vi "Test_Read.vi"   [LabVIEW 2019, in "Test_Maui.Config.lvclass"]
uses:
  Test_Maui.Config.lvclass
  lvsrc/Maui 1.0/Maui.Config/Maui.Config.lvclass
  <vilib>/addons/_JKI Toolkits/Caraya/classes/Test/Test.lvclass
  <vilib>/addons/_JKI Toolkits/Caraya/classes/Assert/Assert.lvclass
  <vilib>/addons/_JKI Toolkits/Caraya/classes/Assert/Assert True.vi
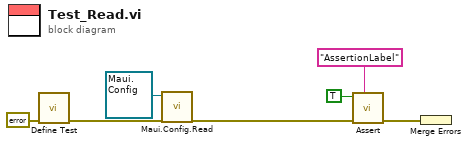
[diagram p0: block diagram]
diagram:
  n1 = call <vilib>:"Define Test.vi"("error in (no error)"=errorcluster {"status"=FALSE, "code"=0, "source"=""}) -> ("error out"=w3:errorcluster)  [unwired: 10 in]
  n2 = call "Maui.Config.Read.vi"("error in (no error)"=w3, "Maui.Config in"=refnum<class "Maui.Config.lvclass"> refnum) -> ("error out"=w2:errorcluster)  [unwired: 7 in, 2 out]
  n3 = call-poly <vilib>:"Assert.vi"("Label"="AssertionLabel" ("Label (VI Title)"), "error in (no error)"=w2, "True?"=TRUE) -> ("error out"=w5:errorcluster)  [unwired: 8 in]
  n4 = Merge Errors(w5) -> ()  [unwired: 1 out]
